vi "connect to FPGA analogue stream.vi"(6 "Data":T1={"Parameters"={"FPGA Ref"=refnum, "data stream"={"data writer name"="error writer", "NS write buffer size"=16, "NS Buffer length"=0}, "FIFO Depth"=0, "Channel controls"={"FIFO channel count"=0, "active indices"=[], "active channels"=0, "channelScaling"=[], "scanivalveCount"=0, "channels"=[]}, "safetyChannels"={"oilP"=0, "airP"=0, "water"=0, "channelLimits"=[]}, "speedChannel"=0, "maxSpeedLimit"=0.0, "Torque"={"fixedOffset"=0.0, "filter"=FALSE, "fallingEdge"=FALSE, "swapEncoders"=FALSE}}, "Variables"={"Intermediary buffer"=[], "buffer position"=0, "write loop counter"=0, "NS write trigger"=0, "NS Connection status"=FALSE, "waiting for NS"=FALSE, "labAmbient"={"pressure"=0.0, "temperature"=0.0}, "scanivalvePorts"=[], "scanivalvePressures"=[], "data stream"="", "activeChannelLimitIndex"=[], "runningSpeedLimit"=0.0, "speedChannelIndex"=0, "Interlocks"={"gearboxOil"=FALSE, "bearingOil"=FALSE, "gearboxAir"=FALSE}, "interlockChannels"={"gearboxOil"=0, "bearingOil"=0, "air"=0}, "limitStates"=[]}}, 11 "RT Queues":T8) -> ()   [LabVIEW 2018]
uses:
  Type Defs/Queues cluster.ctl
  ICL-LabVIEW_General/Message Scheduler/message scheduler.lvclass
  Type Defs/Data processing loop data.ctl
  Type Defs/FPGA reference.ctl
  PC/type defs/channelControl.ctl
  Type Defs/channelScalingTypes.ctl
  Type Defs/scalingMethods.ctl
  ICL-LabVIEW_General/data channels/parent class/Data Channel.lvclass
  PC/type defs/channelLimitControl.ctl
  PC/type defs/limitActions.ctl
  <vilib>/LabVIEW Targets/FPGA/cRIO/shared/nicrio_ModuleControls/nicrio_cRIO-9237_DataRatesRing.ctl
  <vilib>/FPGAPlugInAG/cRIO-9056/niLvFpga_Reset_cRIO-9056.vi
  <vilib>/FPGAPlugInAG/cRIO-9056/niLvFpga_Run_cRIO-9056.vi
  <vilib>/Utility/error.llb/Error Cluster From Error Code.vi
  <vilib>/rvi/errors/niLvFpgaAdjustHostInterfaceError.vi
  <vilib>/rvi/interface/common/niFpgaWaitOnOcc.vi
  <vilib>/rvi/interface/nirviMethod/nirviMethod.xnode
  FPGA Bitfiles/CompressorRigV2_CompressorFPGA_FPGAMainV3_7sPRekuravM.lvbitx
  <vilib>/rvi/interface/nirviReadWriteControl/nirviReadWriteControl.xnode
  <vilib>/ErrorRing/Error Ring.xnode
  <vilib>/rvi/errors/niLvFpgaMergeErrorWithErrorCode.vi
  NiFpgaLv.dll
  <vilib>/FPGAPlugInAG/cRIO-9056/niLvFpga_ReadFifo_cRIO-9056.vi
  <vilib>/FPGAPlugInAG/cRIO-9056/niLvFpga_StopFifo_cRIO-9056.vi
  <vilib>/FPGAPlugInAG/cRIO-9056/niLvFpga_ConfigureFifo_cRIO-9056.vi
panel:
  out "Actual Depth":u32
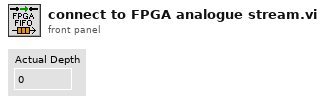
[diagram p1: front panel]
types:
  T1 = typedef "Data processing loop data.ctl" = cluster{"Parameters":cluster{"FPGA Ref":T2, "data stream":cluster{"data writer name":string, "NS write buffer size":i32, "NS Buffer length":u32}, "FIFO Depth":u32, "Channel controls":cluster{"FIFO channel count":i32, "active indices":i16[], "active channels":i32, "channelScaling":T3[], "scanivalveCount":i32, "channels":refnum<class "Data Channel.lvclass">[]}, "safetyChannels":cluster{"oilP":u16, "airP":u16, "water":u16, "channelLimits":T6[]}, "speedChannel":i32, "maxSpeedLimit":dbl, "Torque":cluster{"fixedOffset":dbl, "filter":bool, "fallingEdge":bool, "swapEncoders":bool}}, "Variables":cluster{"Intermediary buffer":dbl[][], "buffer position":u32, "write loop counter":u16, "NS write trigger":u32, "NS Connection status":bool, "waiting for NS":bool, "labAmbient":cluster{"pressure":dbl, "temperature":dbl}, "scanivalvePorts":u16[], "scanivalvePressures":dbl[], "data stream":refnum<k21>, "activeChannelLimitIndex":u16[], "runningSpeedLimit":dbl, "speedChannelIndex":i32, "Interlocks":cluster{"gearboxOil":bool, "bearingOil":bool, "gearboxAir":bool}, "interlockChannels":cluster{"gearboxOil":i32, "bearingOil":i32, "air":i32}, "limitStates":cluster{"warn":bool, "alarm":bool}[]}}
  T2 = typedef "FPGA reference.ctl" = refnum<k20>
  T3 = typedef "channelControl.ctl" = cluster{"index":u16, "active":bool, "channelType":T4, "module":u16, "terminal":u16, "channelName":string, "scalingMethod":T5, "scalingParameters":dbl[], "scaledUnits":string, "tempOffset":dbl}
  T4 = typedef "channelScalingTypes.ctl" = enum16{"calculation", "measurement", "scanivalve", "output", "digital"}
  T5 = typedef "scalingMethods.ctl" = enum16{"none", "linear", "thermocouple", "polynomial", "encoder", "RTD"}
  T6 = typedef "channelLimitControl.ctl" = cluster{"channelID":u16, "Enabled":bool, "warnValue":dbl, "limitValue":dbl, "Invert":bool, "limitAction":T7}
  T7 = typedef "limitActions.ctl" = enum16{"stop", "shutdown", "ignore"}
  T8 = typedef "Queues cluster.ctl" = cluster{"RT Message":refnum<queue>, "RT Comms":refnum<queue>, "RT Data":refnum<queue>, "RT FIFO":refnum<queue>, "message scheduler":refnum<class "message scheduler.lvclass">}
  T9 = cluster{"filterSize":u8, "lowerThreshold":u8, "upperThreshold":u8}
  T10 = typedef "nicrio_cRIO-9237_DataRatesRing.ctl" = u8
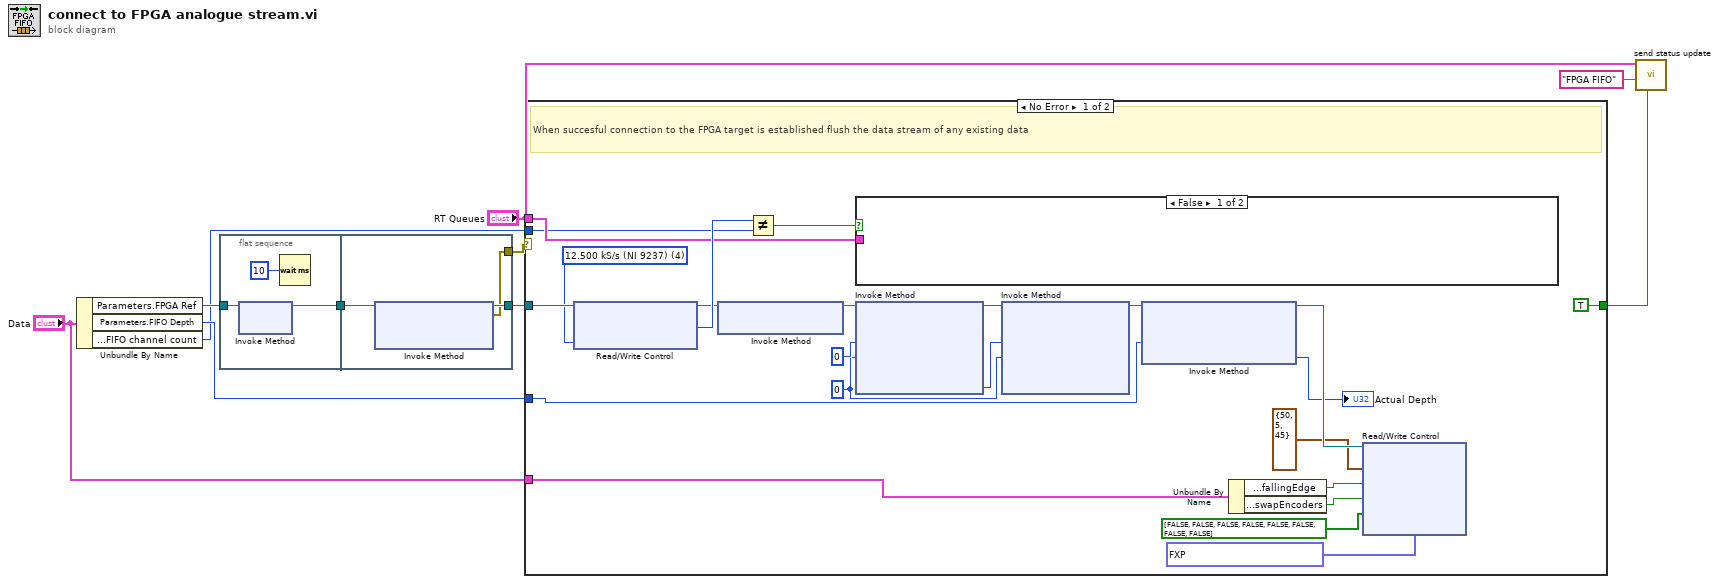
[diagram p0: block diagram]
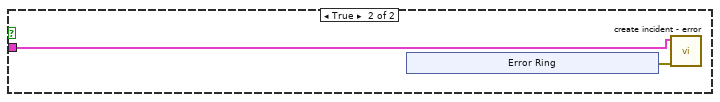
[diagram p2: hidden frame]
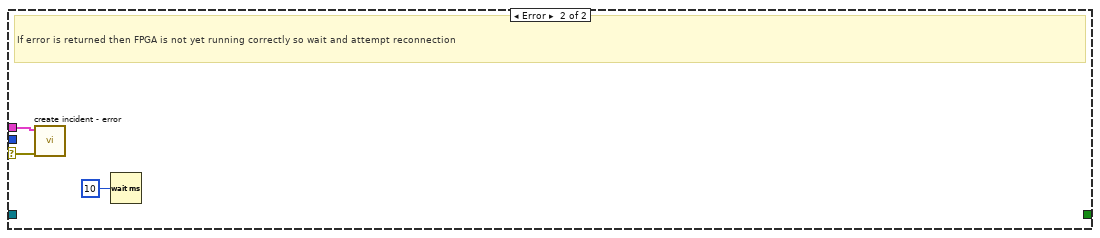
[diagram p3: hidden frame]
diagram:
  n1 = Unbundle By Name("Data") -> ("Parameters.FPGA Ref"=w10:T2, "Parameters.FIFO Depth"=w5:u32, "Parameters.Channel controls.FIFO channel count"=w4:i32)
  n2 = flat-sequence {
    tunnel: w10 -> [w13]
    tunnel: [w12] -> w3
    tunnel: [w15] -> w9
    tunnel: w3 -> [w16]
    tunnel: [w14] -> w2
    frame #0 {
      n3 = xnode "Invoke Method"("FPGA VI Reference In"=w13) -> ("FPGA VI Reference Out"=w12:T2)  [unwired: 1 in, 1 out]
      n4 = Wait (ms)(milliseconds to wait=u32 10) -> ()  [unwired: 1 out]
    }
    frame #1 {
      n5 = xnode "Invoke Method"("FPGA VI Reference In"=w16) -> ("FPGA VI Reference Out"=w15:T2, "error out"=w14:errorcluster)  [unwired: 2 in]
    }
  }
  n6 = case shown="No Error" w2 {
    selector: w2 -> [_ w48]
    tunnel: w9 -> [w33 _]
    tunnel: [TRUE _] -> w7
    tunnel: "RT Queues" -> [w29 w47]
    tunnel: w5 -> [w31 _]
    tunnel: w4 -> [w28 _]
    tunnel: "Data" -> [w22 _]
    frame No Error {
      w23 = T10 4 items=["50.000 kS/s (NI 9237)"=1, "25.000 kS/s (NI 9237)"=2, "16.667 kS/s (NI 9237)"=3, "12.500 kS/s (NI 9237)"=4, "10.000 kS/s (NI 9237)"=5, "8.333 kS/s (NI 9237)"=6, "7.143 kS/s (NI 9237)"=7, "6.250 kS/s (NI 9237)"=8, "5.556 kS/s (NI 9237)"=9, "5.000 kS/s (NI 9237)"=10, "4.545 kS/s (NI 9237)"=11, "4.167 kS/s (NI 9237)"=12, "3.846 kS/s (NI 9237)"=13, "3.571 kS/s (NI 9237)"=14, "3.333 kS/s (NI 9237)"=15, "3.125 kS/s (NI 9237)"=16, "2.941 kS/s (NI 9237)"=17, "2.778 kS/s (NI 9237)"=18, "2.632 kS/s (NI 9237)"=19, "2.500 kS/s (NI 9237)"=20, "2.381 kS/s (NI 9237)"=21, "2.273 kS/s (NI 9237)"=22, "2.174 kS/s (NI 9237)"=23, "2.083 kS/s (NI 9237)"=24, "2.000 kS/s (NI 9237)"=25, "1.923 kS/s (NI 9237)"=26, "1.852 kS/s (NI 9237)"=27, "1.786 kS/s (NI 9237)"=28, "1.724 kS/s (NI 9237)"=29, "1.667 kS/s (NI 9237)"=30, "1.613 kS/s (NI 9237)"=31] ("Data Rate")
      w36 = 0 ("Timeout (ms)")
      # "When succesful connection to the FPGA target is established flush the data stream of any existing data"
      n7 = xnode "Read/Write Control"("FPGA VI Reference In"=w33, "Data Rate"=w23) -> ("FPGA VI Reference Out"=w25:T2, "Total channel count"=w32:u32)  [unwired: 1 in, 1 out]
      n8 = xnode "Invoke Method"("FPGA VI Reference In"=w25) -> ("FPGA VI Reference Out"=w24:T2)  [unwired: 1 in, 1 out]
      n9 = Not Equal?(x=w32, y=w28) -> (x != y?=w30:bool)
      n10 = case shown="False" w30 {
        tunnel: w29 -> [_ w41]
        frame False {
        }
        frame True {
          n11 = xnode "Error Ring"() -> ("error out"=w40:errorcluster)
          n12 = call "create incident - error.vi"("error"=w40, "RT Queues"=w41) -> ()  [unwired: 9 in, 1 out]
        }
      }
      n13 = xnode "Invoke Method"("FPGA VI Reference In"=w24, "Number of Elements"=u32 0, "Timeout (ms)"=w36) -> ("FPGA VI Reference Out"=w38:T2, "Elements Remaining"=w37:u32)  [unwired: 1 in, 2 out]
      n14 = xnode "Invoke Method"("FPGA VI Reference In"=w38, "Number of Elements"=w37, "Timeout (ms)"=w36) -> ("FPGA VI Reference Out"=w34:T2)  [unwired: 1 in, 3 out]
      n15 = xnode "Invoke Method"("FPGA VI Reference In"=w34, "Requested Depth"=w31) -> ("FPGA VI Reference Out"=w27:T2, "Actual Depth"=→"Actual Depth":u32)  [unwired: 1 in, 1 out]
      n16 = Unbundle By Name(w22) -> ("Parameters.Torque.fallingEdge"=w21:bool, "Parameters.Torque.swapEncoders"=w20:bool)
      n17 = xnode "Read/Write Control"("FPGA VI Reference In"=w27, "Edge filter"=T9 {"filterSize"=50, "lowerThreshold"=5, "upperThreshold"=45}, "falling edge (F)"=w21, "switch encoders"=w20, "Safe Digital"=bool[] [FALSE, FALSE, FALSE, FALSE, FALSE, FALSE, FALSE, FALSE], "Safe Voltage"=fxp<+/-,20,5>[] [0.0, 0.0, 0.0, 0.0]) -> ()  [unwired: 1 in, 2 out]
    }
    frame Error {
      # "If error is returned then FPGA is not yet running correctly so wait and attempt reconnection"
      n18 = call "create incident - error.vi"("error"=w48, "RT Queues"=w47) -> ()  [unwired: 9 in, 1 out]
      n19 = Wait (ms)(milliseconds to wait=u32 10) -> ()  [unwired: 1 out]
    }
  }
  n20 = call "send status update.vi"("status (F)"=w7, "subject"="FPGA FIFO" ("Message"), "RT Queues"="RT Queues") -> ()  [unwired: 8 in, 1 out]
